vi "Create_Object.vi"(8 "error in (no error)":errorcluster, 9 "Terminal Map in":map{string, T1}(c390), 10 "owner refnum":variant, 11 "Control in":refnum<class "Control.lvclass">) -> (0 "error out":errorcluster, 1 "Terminal Map Out":map{string, T1}(c390), 3 "Control out":refnum<class "Control.lvclass">)   [LabVIEW 2025, in "Control.lvclass"]
uses:
  Control.lvclass
  C:/Users/mrjak/Documents/GitHub/LVGPT/LabVIEW/VIs/Classes/Node/Node.lvclass
  Terminal.ctl
  Node.lvclass/Node.ctl
  Node.lvclass
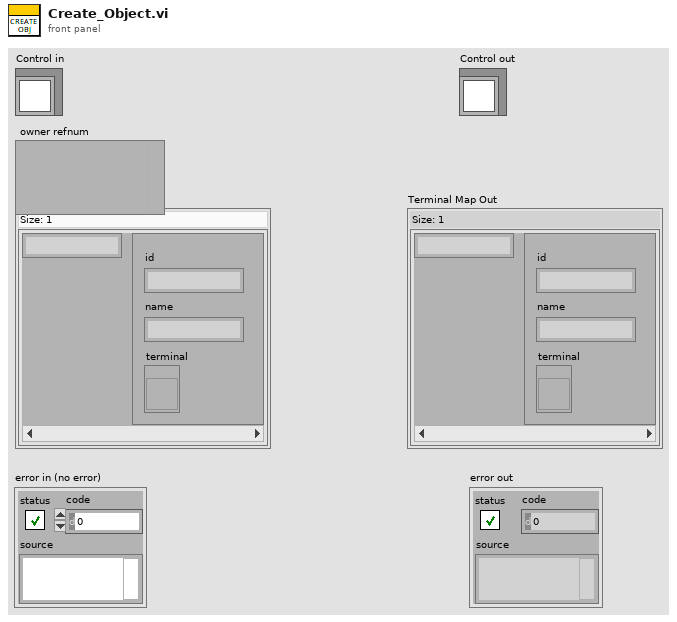
[diagram p1: front panel]
types:
  T1 = typedef "Terminal.ctl" = cluster{"id":string, "name":string, "terminal":refnum<vi>}
  T2 = typedef "LVPointTypeDef.ctl" = cluster{"Horizontal":i16, "Vertical":i16}
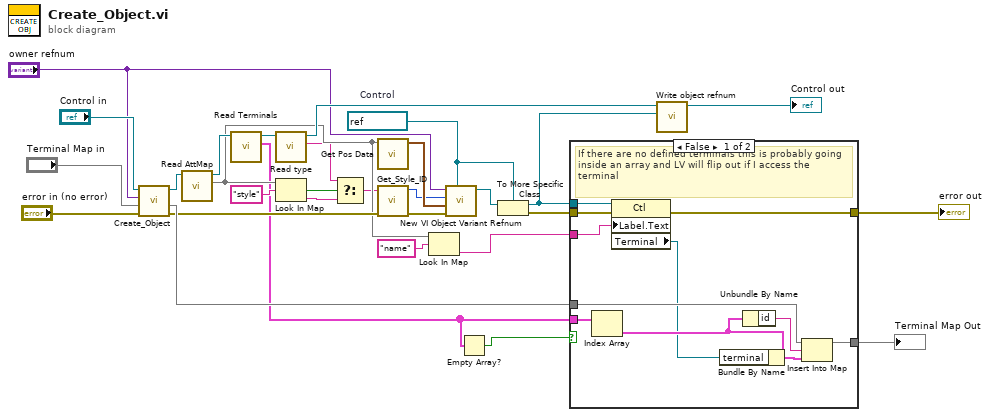
[diagram p0: block diagram]
diagram:
  w5 = refnum<vi> refnum  # Control
  n1 = call-parent "Create_Object.vi"("error in (no error)"="error in (no error)", "Terminal Map in"="Terminal Map in", "owner refnum"="owner refnum", "Node in"="Control in") -> ("error out"=w18:errorcluster, "Terminal Map Out"=w19:map{string, T1}, "Node out"=w20:refnum<class "Control.lvclass">)  [unwired: 5 in]
  n2 = call "Read AttMap.vi"("Node in"=w20) -> ("AttMap"=w13:map{string, string}, "Node out"=w27:refnum<class "Control.lvclass">)  [unwired: 8 in, 1 out]
  n3 = call "Read Terminals.vi"("Node in"=w27) -> ("Terminals"=w8:T1[], "Node out"=w26:refnum<class "Control.lvclass">)  [unwired: 8 in, 1 out]
  n4 = call "Read type.vi"("Node in"=w26) -> ("type"=w11:string, "Node out"=w17:refnum<class "Control.lvclass">)  [unwired: 8 in, 1 out]
  n5 = Look In Map(map=w13, key="style") -> (key not found?=w12:bool, value=w10:string)  [unwired: 1 in]
  n6 = Select(t=w11, s=w12, f=w10) -> (s? t:f=w9:string)
  n7 = call "Get Pos Data.vi"("AttMap"=w13) -> ("Position"=w24:T2)  [unwired: 10 in]
  n8 = call "Get_Style_ID.vi"("error in (no error)"=w18, "Style"=w9) -> ("error out"=w22:errorcluster, "style"=w23:i32)  [unwired: 7 in, 1 out]
  n9 = Look In Map(map=w13, key="name") -> (value=w1:string)  [unwired: 1 in, 1 out]
  n10 = call "New VI Object Variant Refnum.vi"("vi object class"=w5, "error in (no error)"=w22, "location"=w24, "style"=w23, "owner refnum"="owner refnum") -> ("object refnum"=w21:refnum<vi>)  [unwired: 5 in, 1 out]
  n11 = Empty Array?(array=w8) -> (empty?=w7:bool)
  n12 = To More Specific Class(target class=w5, reference=w21) -> (specific class reference=w3:refnum<vi>, error out=w4:errorcluster)  [unwired: 1 in]
  n13 = case shown="False" w7 {
    tunnel: w19 -> [w38 w43]
    tunnel: [w37 w43] -> w15
    tunnel: w8 -> [w36 _]
    tunnel: w4 -> [w35 w42]
    tunnel: w3 -> [w34 _]
    tunnel: [w33 w42] -> w2
    tunnel: w1 -> [w32 _]
    frame False {
      # "If there are no defined terminals this is probably going inside an array and LV will flip out if I access the terminal"
      n14 = Index Array(array=w36) -> (element=w40:T1)  [unwired: 1 in]
      n15 = property class="Ctl"(reference=w34, error in=w35, "Label.Text"=w32) -> (error out=w33:errorcluster, "Terminal"=w31:refnum<vi>)  [unwired: 1 out]
      n16 = Bundle By Name(cluster=w40, "terminal"=w31) -> (w39:T1)
      n17 = Unbundle By Name(w40) -> ("id"=w41:string)
      n18 = Insert Into Map(map in=w38, key=w41, value=w39) -> (map out=w37:map{string, T1})  [unwired: 2 out]
    }
    frame True {
    }
  }
  "error out" <- w2
  "Terminal Map Out" <- w15
  n19 = call-dynamic "Write object refnum.vi"("object refnum"=w3, "Node in"=w17) -> ("Node out"=→"Control out":refnum<class "Control.lvclass">)  [unwired: 8 in, 1 out]
